vi "BU-UCFParsing.vi"() -> (3 "Gate values":string[][](table))   [LabVIEW 2014]
panel:
  out "n":string[](array[string])
  out "K":string[](array[string])
  out "ymin":string[](array[string])
  out "ymax":string[](array[string])
  out "Gate Names":string[](array[string])
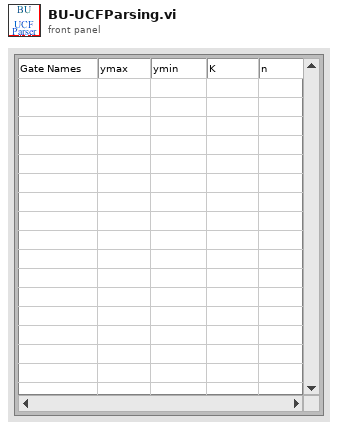
[diagram p1: front panel]
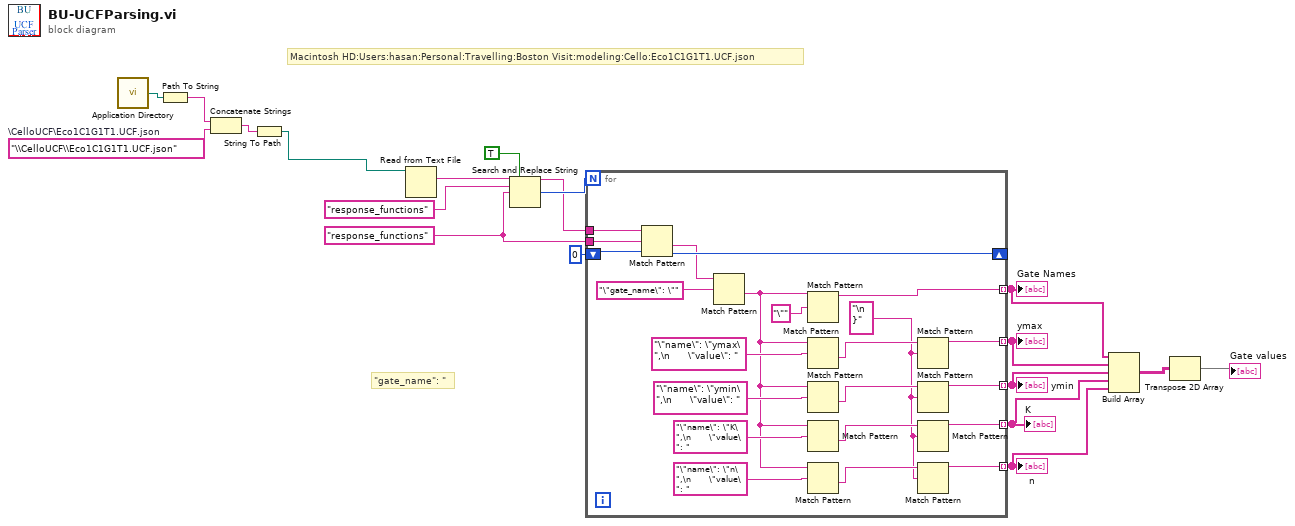
[diagram p0: block diagram]
diagram:
  w3 = "\\CelloUCF\\Eco1C1G1T1.UCF.json"  # \CelloUCF\Eco1C1G1T1.UCF.json
  w13 = "response_functions" ("search string")
  # "\"gate_name\": \""
  # "Macintosh HD:Users:hasan:Personal:Travelling:Boston Visit:modeling:Cello:Eco1C1G1T1.UCF.json"
  n1 = call <vilib>:"Application Directory.vi"() -> ("Application Directory"=w5:path)
  n2 = Path To String(path=w5) -> (string=w4:string)
  n3 = Concatenate Strings(w4, w3) -> (w2:string)
  n4 = String To Path(string=w2) -> (path=w1:path)
  n5 = Read from Text File(file (use dialog)=w1) -> (text=w19:string)  [unwired: 3 in, 3 out]
  n6 = Search and Replace String(replace all?=TRUE ("replace all? (F)"), input string=w19, search string="response_functions", replace string=w13) -> (result string=w15:string, number of replacements=w16:i32)  [unwired: 4 in, 2 out]
  n7 = for {
    N: w16 -> [_]
    tunnel: w15 -> [w41]
    shift-right: [w39] -> _
    shift-left: 0 ("offset past match") -> [w40]
    tunnel: w13 -> [w38]
    tunnel: [w34] -> w12 mode=indexing
    tunnel: [w23] -> w11 mode=indexing
    tunnel: [w22] -> w10 mode=indexing
    tunnel: [w21] -> w9 mode=indexing
    tunnel: [w20] -> w8 mode=indexing
    w24 = "\n    }" ("search string")
    n8 = Match Pattern(string=w41, regular expression=w38, offset (0)=w40) -> (after substring=w37:string, offset past match=w39:i32)  [unwired: 2 out]
    n9 = Match Pattern(string=w37, regular expression="\"gate_name\": \"" ("search string")) -> (after substring=w29:string)  [unwired: 1 in, 3 out]
    n10 = Match Pattern(string=w29, regular expression="\"" ("search string")) -> (before substring=w34:string)  [unwired: 1 in, 3 out]
    n11 = Match Pattern(string=w29, regular expression="\"name\": \"ymax\",\n      \"value\": " ("search string")) -> (after substring=w28:string)  [unwired: 1 in, 3 out]
    n12 = Match Pattern(string=w29, regular expression="\"name\": \"ymin\",\n      \"value\": " ("search string")) -> (after substring=w27:string)  [unwired: 1 in, 3 out]
    n13 = Match Pattern(string=w29, regular expression="\"name\": \"K\",\n      \"value\": " ("search string")) -> (after substring=w26:string)  [unwired: 1 in, 3 out]
    n14 = Match Pattern(string=w29, regular expression="\"name\": \"n\",\n      \"value\": " ("search string")) -> (after substring=w25:string)  [unwired: 1 in, 3 out]
    n15 = Match Pattern(string=w28, regular expression=w24) -> (before substring=w23:string)  [unwired: 1 in, 3 out]
    n16 = Match Pattern(string=w27, regular expression=w24) -> (before substring=w22:string)  [unwired: 1 in, 3 out]
    n17 = Match Pattern(string=w26, regular expression=w24) -> (before substring=w21:string)  [unwired: 1 in, 3 out]
    n18 = Match Pattern(string=w25, regular expression=w24) -> (before substring=w20:string)  [unwired: 1 in, 3 out]
  }
  "Gate Names" <- w12
  "ymax" <- w11
  "ymin" <- w10
  "K" <- w9
  "n" <- w8
  n19 = Build Array(w12, w11, w10, w9, w8) -> (w7:string[][])
  n20 = Transpose 2D Array(2D array=w7) -> (transposed array=→"Gate values":string[][])
